vi "Get Item by name.vi"(8 "error in (no error)":errorcluster, 10 "name":string, 11 "JSON Value In":refnum<class "JSON Value.lvclass">) -> (0 "error out":errorcluster, 1 "found":bool, 2 "Value":refnum<class "JSON Value.lvclass">, 3 "JSON Value Out":refnum<class "JSON Value.lvclass">)   [LabVIEW 2020, in "Library Commun.lvlib" / "JSON Value.lvclass"]
doc: "Gets a <b>JSON Value</b> from a JSON collection by <b>name</b>.\n\nCopyright 2012 James David Powell, Shaun Rumbell and Ton Plomp\nMore information on http://lavag.org/topic/16217-cr-json-labview"
uses:
  JSON Value.lvclass
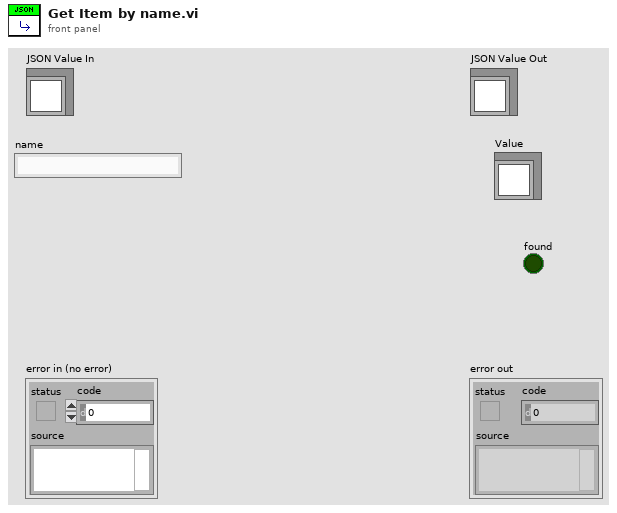
[diagram p1: front panel]
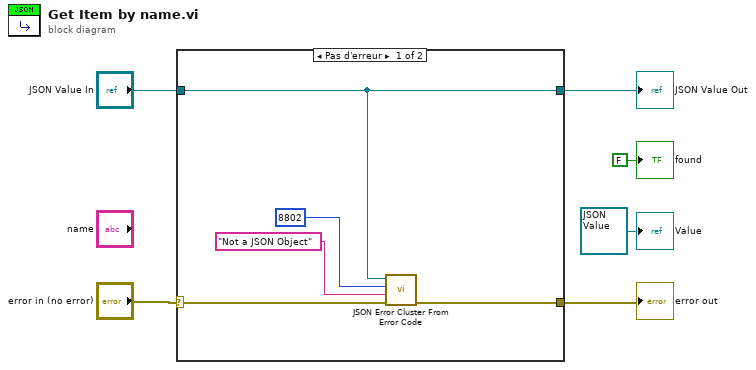
[diagram p0: block diagram]
diagram:
  n1 = case shown="Pas d'erreur" "error in (no error)" {
    selector: "error in (no error)" -> [w9 w13]
    tunnel: [w10 w13] -> w5
    tunnel: [w11 w12] -> w4
    tunnel: "JSON Value In" -> [w11 w12]
    frame No Error {
      n2 = call "JSON Error Cluster From Error Code.vi"("error in (no error)"=w9, "Error message"="Not a JSON Object", "JSON error code"=8802, "JSON Value in"=w11) -> ("error out"=w10:errorcluster)  [unwired: 6 in, 1 out]
    }
    frame Error {
    }
  }
  "error out" <- w5
  "JSON Value Out" <- w4
  "found" <- FALSE ("found")
  "Value" <- refnum<class "JSON Value.lvclass"> refnum ("Value")
